vi "Laser_PM_FPGA.vi"() -> ()   [LabVIEW 2019]
uses:
  <vilib>/rvi/Emulation/niFpgaGetClockAttributes.vi
  <vilib>/rvi/Emulation/niFpgaSctlEmulationGetInTimedLoop.vi
  <vilib>/rvi/Emulation/niFpgaEmulationReportErrorSimple.vi
  <vilib>/rvi/eio/common/nirviEmuTemplateMethod_errors.vi
  <vilib>/rvi/DataTransferAndStorage/Container/Common/niFpgaContainerExecOnDevCompGetState.vi
  <vilib>/rvi/Emulation/niFpgaEmulationIsFPGAContextNoSignature.vi
  <vilib>/rvi/errors/niFpgaSetErrorForExecOnDevCompSimple.vi
  <vilib>/rvi/eio/common/nirviEmuReportErrorAndStop.vi
  <vilib>/rvi/DataTransferAndStorage/Container/Common/niFpgaContainerGetUniqueNameForEmu.vi
  <vilib>/rvi/FIFO/Fifo_Resource/nirvififoEmulationSetSize.vi
  <vilib>/rvi/FIFO/Fifo_Resource/nirviFifoEmulationQueueMgr.vi
  <instcachedir>/0/nirviFifoEmulationQueueMgr_E5CAEC123FF24DC58D834DCA3CDAA9B5.lvgen/nirviFifoEmulationQueueMgr_E5CAEC123FF24DC58D834DCA3CDAA9B5_000.vi
  <vilib>/rvi/FIFO/Fifo_Resource/nirvififoEmulationDetermineInputValidOut.vi
  <vilib>/rvi/FIFO/Fifo_Resource/nirvififoEmulationCreateLock.vi
  <vilib>/rvi/Emulation/niFpgaProcessEmulError.vi
  <vilib>/rvi/FIFO/Fifo_Resource/nirvififoEmulationObtainLock.vi
  <vilib>/rvi/FIFO/Fifo_Resource/nirvififoEmulationReleaseLock.vi
  <vilib>/rvi/occurrence/nirviWaitOnOccurrenceBase.vi
  <vilib>/rvi/errors/nirviReportUnexpectedCaseInternalError.vi
  <vilib>/rvi/errors/nirviReportUnexpectedCaseInternalError (U32).vi
  <vilib>/Utility/error.llb/Clear Errors.vi
  <vilib>/rvi/interface/RandomDataEmulation/niFpgaRandomDataHandleErrors.vi
  <instcachedir>/0/nirviFifoEmulationQueueMgr_E5CAEC123FF24DC58D834DCA3CDAA9B5.lvgen/nirviFifoEmulationQueueMgr_E5CAEC123FF24DC58D834DCA3CDAA9B5_001.vi
  <vilib>/rvi/Emulation/niFpgaCriticalErrorInLSC.vi
  <vilib>/eio/EIONode/EIONode.xnode
  <vilib>/rvi/DataTransferAndStorage/Container/XNode/niFpgaContainer.xnode
  <vilib>/rvi/FIFO/Fifo_Resource/niFpgaFifoEmulationRefIn.vi
panel:
  out "Count T/O":bool
  out "Load":u16
  out "laser":i16
  out "Laser T/O":bool
  in  "Timeout":i32
  in  "trigger":bool
  in  "stop":bool
  out "Count":u32 caption="Tick Count(uSec)"
  in  "Count(uSec)":u32
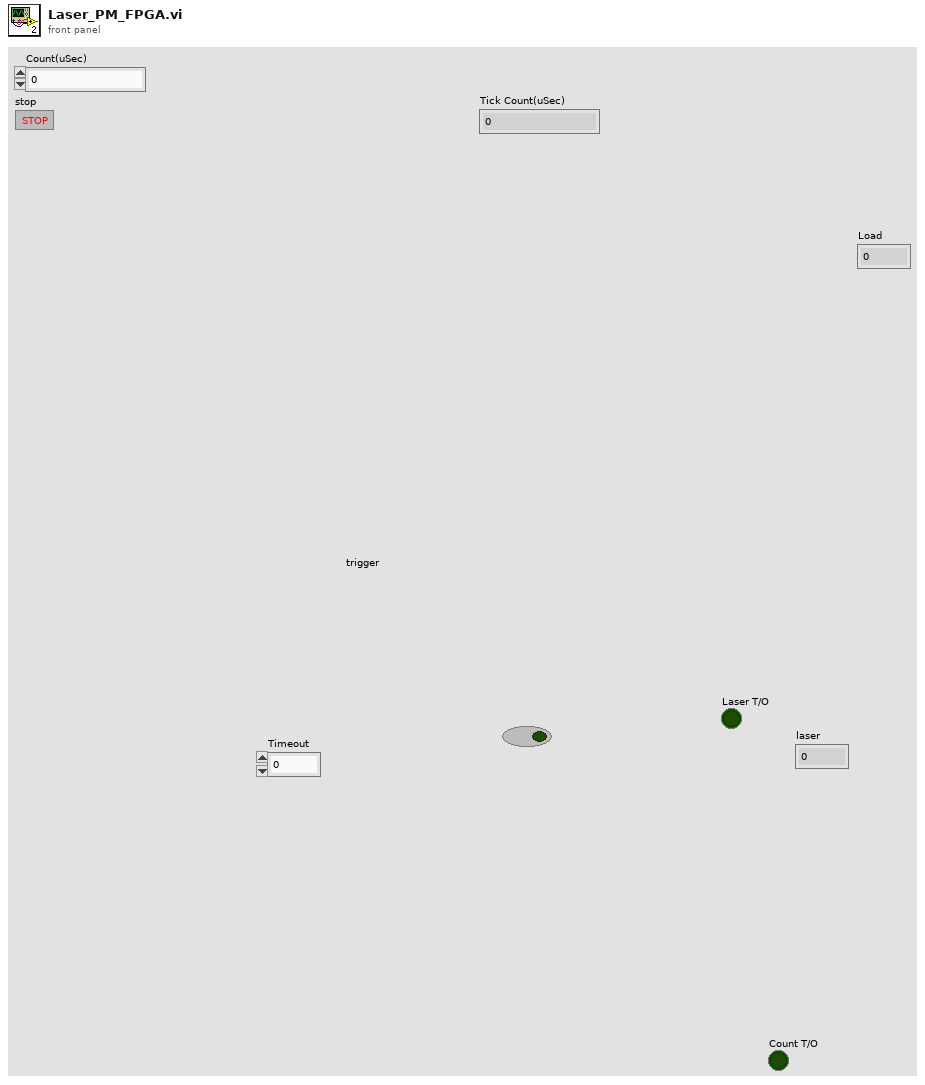
[diagram p1: front panel]
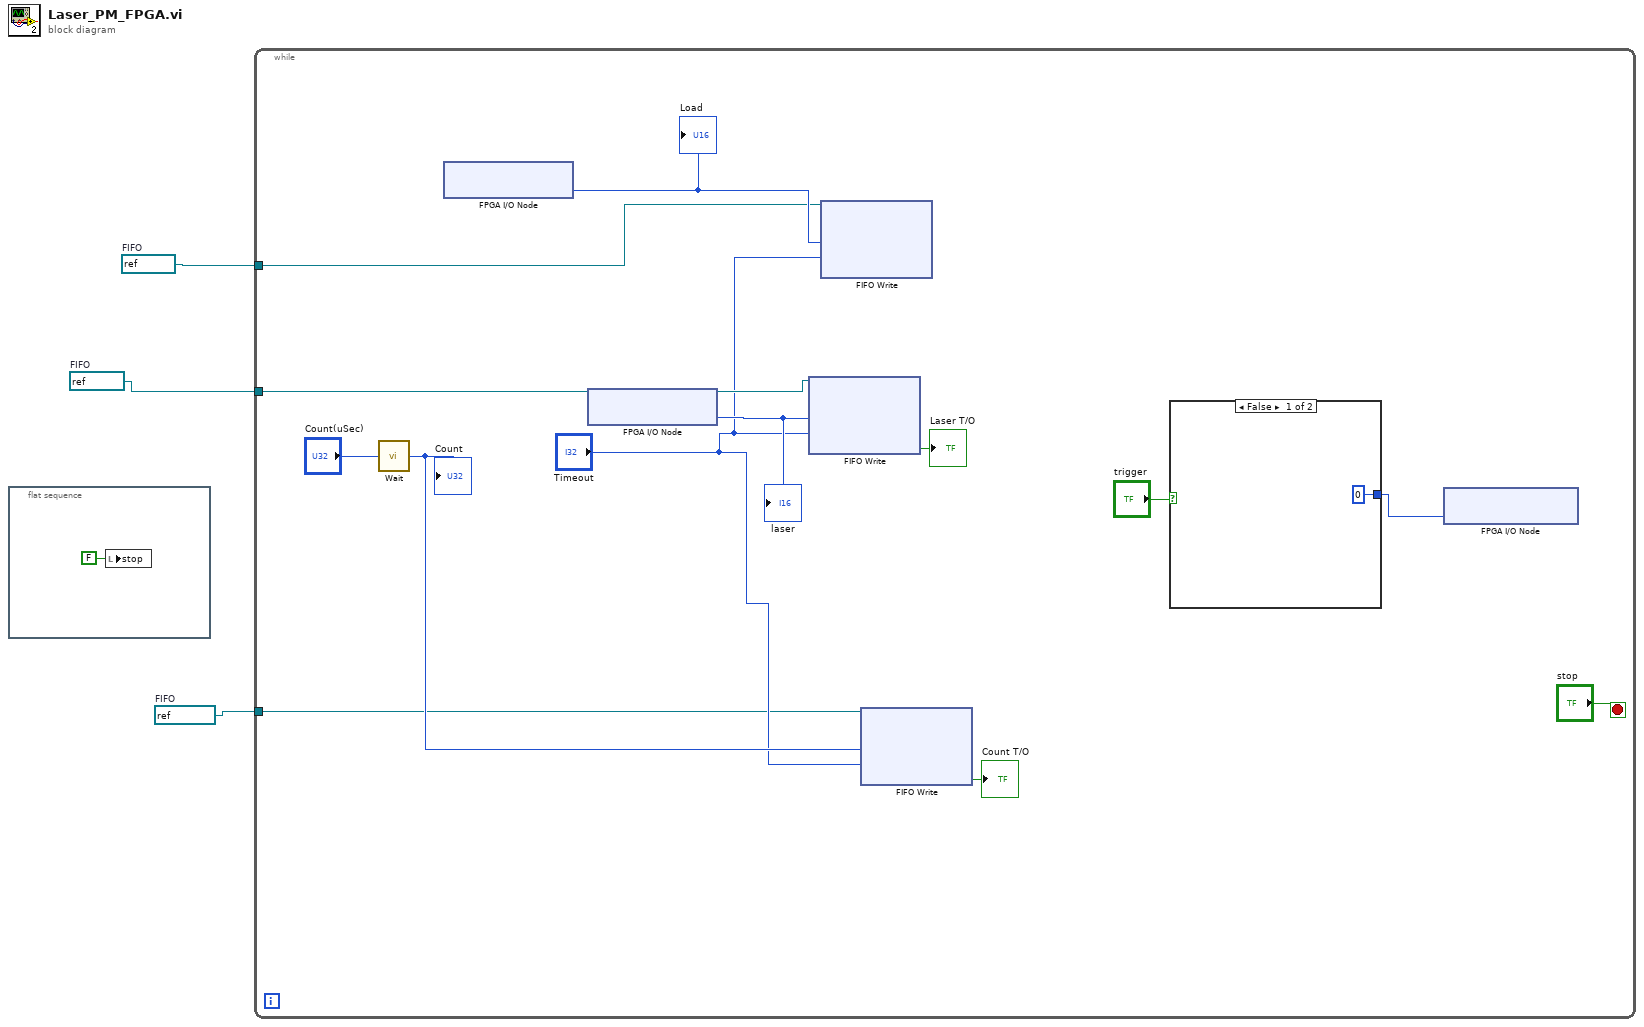
[diagram p0: block diagram]
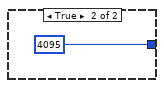
[diagram p2: hidden frame]
diagram:
  w1 = refnum<k21> "Count"  # FIFO
  w2 = refnum<k21> "Load"  # FIFO
  w3 = refnum<k21> "Laser"  # FIFO
  n1 = flat-sequence {
    frame #0 {
      n2 = local write "stop"(FALSE ("stop")) -> ()
    }
  }
  n3 = while {
    tunnel: w3 -> [w11]
    tunnel: w2 -> [w9]
    tunnel: w1 -> [w5]
    stop <- "stop" stop-if-true
    n4 = call "Wait"("Count(uSec)"="Count(uSec)") -> ("Tick Count(uSec)"=w7:u32)
    "Count" <- w7
    n5 = xnode "FPGA I/O Node"() -> ("ConnectorA/AI1"=w10:u16)  [unwired: 1 in, 1 out]
    "Load" <- w10
    n6 = xnode "FPGA I/O Node"() -> ("ConnectorC/AI0"=w12:i16)  [unwired: 1 in, 1 out]
    "laser" <- w12
    n7 = xnode "FIFO Write"("Element"=w12, "Timeout"="Timeout", "FIFO In"=w11) -> ("Timed Out?"=→"Laser T/O":bool)  [unwired: 1 out]
    n8 = xnode "FIFO Write"("Element"=w10, "Timeout"="Timeout", "FIFO In"=w9) -> ()  [unwired: 2 out]
    n9 = xnode "FIFO Write"("Element"=w7, "Timeout"="Timeout", "FIFO In"=w5) -> ("Timed Out?"=→"Count T/O":bool)  [unwired: 1 out]
    n10 = case shown="False" "trigger" {
      tunnel: [u16 0 ("ConnectorA/AO0") u16 4095 ("ConnectorA/AO0")] -> w14
      frame False {
      }
      frame True {
      }
    }
    n11 = xnode "FPGA I/O Node"("ConnectorB/AO0"=w14) -> ()  [unwired: 1 in, 1 out]
  }
